vi "Open Bus Monitor.vi"(8 "error in (no error)":errorcluster, 11 "Mediator in":refnum<class "Mediator.lvclass">) -> (0 "error out":errorcluster, 3 "Mediator out":refnum<class "Mediator.lvclass">)   [LabVIEW 2015, in "Mediator.lvlib" / "Mediator.lvclass"]
uses:
  Mediator.lvclass
  Mediator.lvclass/Mediator.ctl
  IViewable/IViewable/View Position Enum.ctl
  IViewable/IViewable Messages/Open Front Panel Msg/Open Front Panel Msg.lvclass/Open Front Panel Msg.ctl
  <vilib>/ActorFramework/Message Enqueuer/Message Enqueuer.lvclass/Message Enqueuer.ctl
  <vilib>/ActorFramework/Message Enqueuer/Enqueue.vi
  <vilib>/ActorFramework/Message Priority Queue/Priority Enqueue.vi
  <vilib>/ActorFramework/Message Enqueuer/Message Enqueuer.lvclass
  IViewable/IViewable Messages/Open Front Panel Msg/Open Front Panel Msg.lvclass
  IViewable/IViewable/IViewable.lvclass
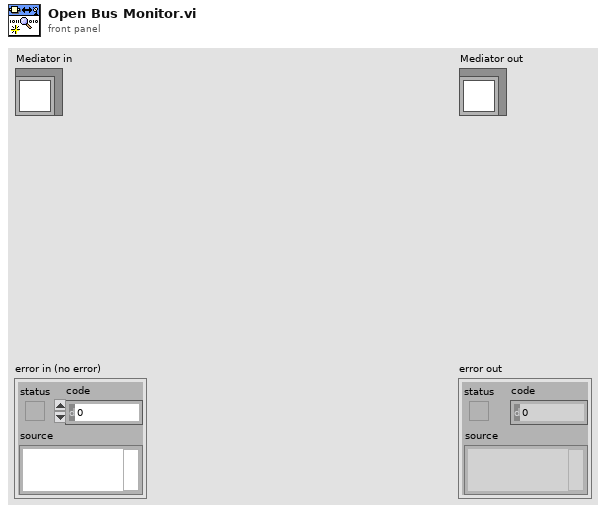
[diagram p1: front panel]
types:
  T1 = typedef "IViewable.lvlib/IViewable.lvclass/View Position Enum.ctl" = enum16{"Centered", "Maximized", "Minimized", "Custom", "Unchanged"}
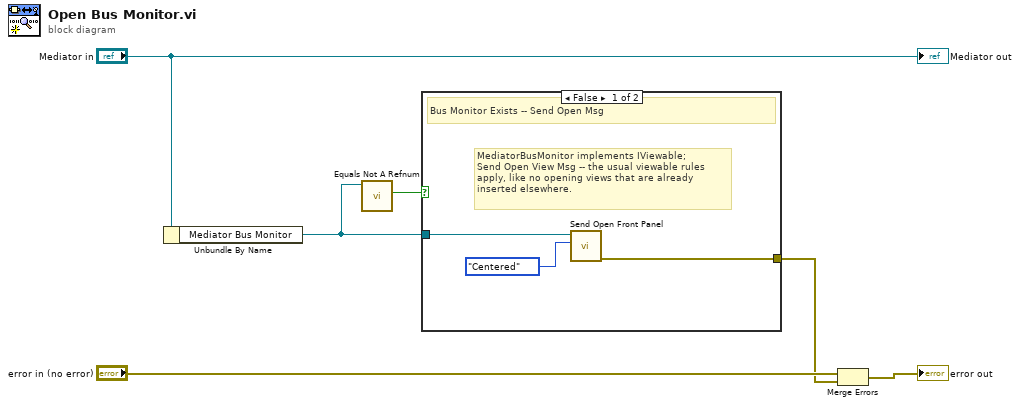
[diagram p0: block diagram]
diagram:
  n1 = Unbundle By Name("Mediator in") -> ("Mediator Bus Monitor"=w2:refnum<class "Message Enqueuer.lvclass">)
  n2 = call <vilib>:"Equals Not A Refnum.vi"("Message Enqueuer"=w2) -> ("Not a refnum?"=w1:bool)  [unwired: 10 in]
  n3 = case shown="False" w1 {
    tunnel: w2 -> [w9 _]
    tunnel: [w8 _] -> w3
    frame False {
      # "MediatorBusMonitor implements IViewable;\nSend Open View Msg -- the usual viewable rules\napply, like no opening views that are already\ninserted elsewhere."
      # "Bus Monitor Exists -- Send Open Msg"
      n4 = call "Send Open Front Panel.vi"("Position"=View_Position_Enum."Centered", "Message Enqueuer"=w9) -> ("error out"=w8:errorcluster)  [unwired: 8 in, 1 out]
    }
    frame True {
      # "No Bus Monitor -- Send nothing"
    }
  }
  n5 = Merge Errors("error in (no error)", w3) -> (→"error out":errorcluster)
  "Mediator out" <- "Mediator in"
